vi "SRS Ramp Aux Voltage.vi"() -> ()   [LabVIEW 2020]
panel:
  in  "Channel #":i32=1 min=1 max=4 step=1
  out "Time Remaining":dbl=60.0 format="%<%H:%M:%S>t"
  out "Output Voltage":dbl format="%_4g"
  in  "Time (Hr:Min:Sec)":dbl=60.0 step=1.0 format="%<%H:%M:%S>t"
  in  "Stop Voltage":dbl=0.01 format="%_4g"
  in  "Start Ramp":bool
  in  "Cycle Time":dbl=0.1 format="%.3g"
  in  "stop":bool
  in  "VISA resource name":refnum<visa-resource-name>
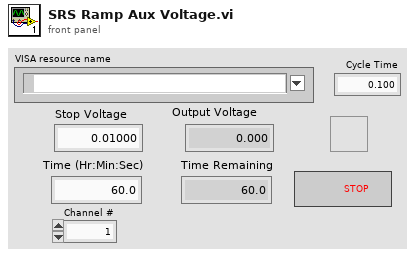
[diagram p1: front panel]
types:
  T1 = enum8{"Enabled", "Disabled", "Disabled and Grayed Out"}
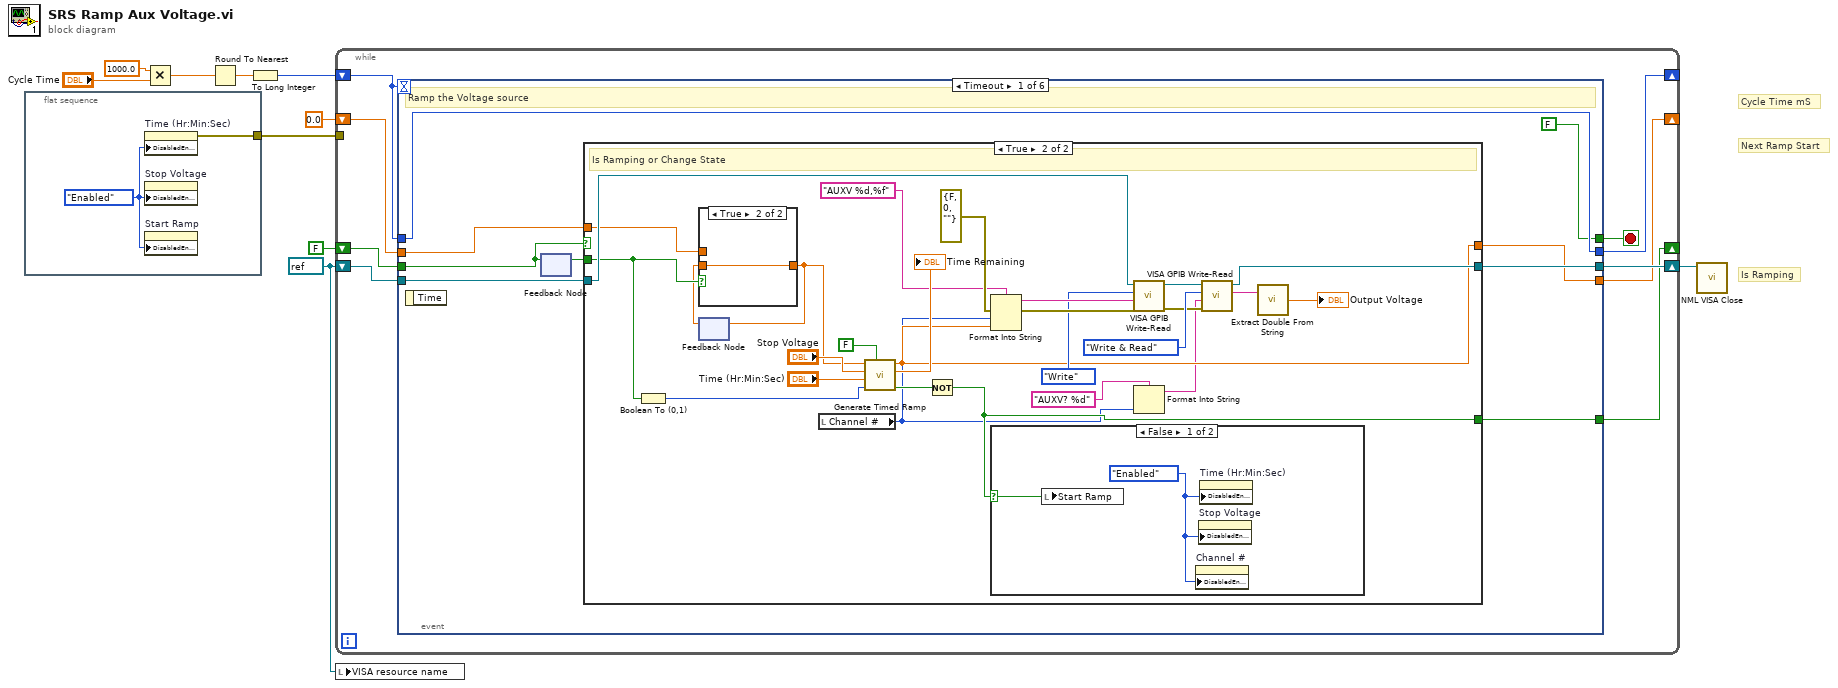
[diagram p0: block diagram]
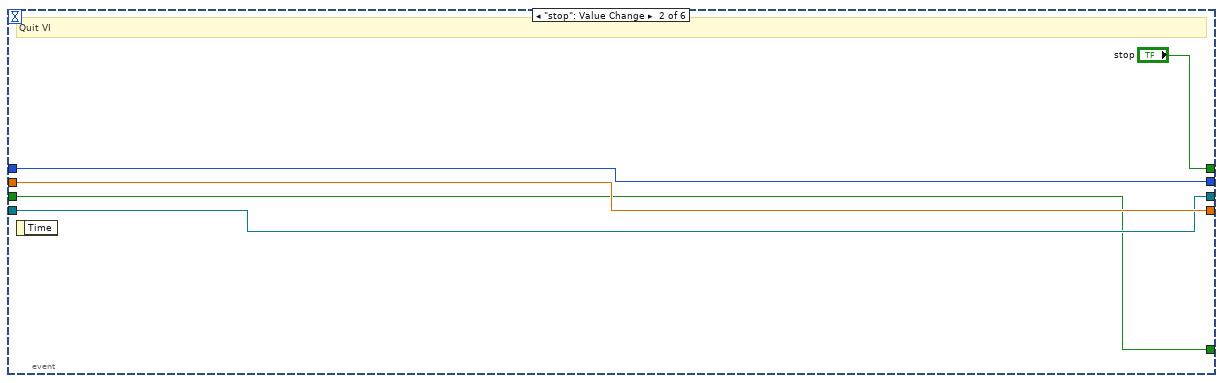
[diagram p5: hidden frame]
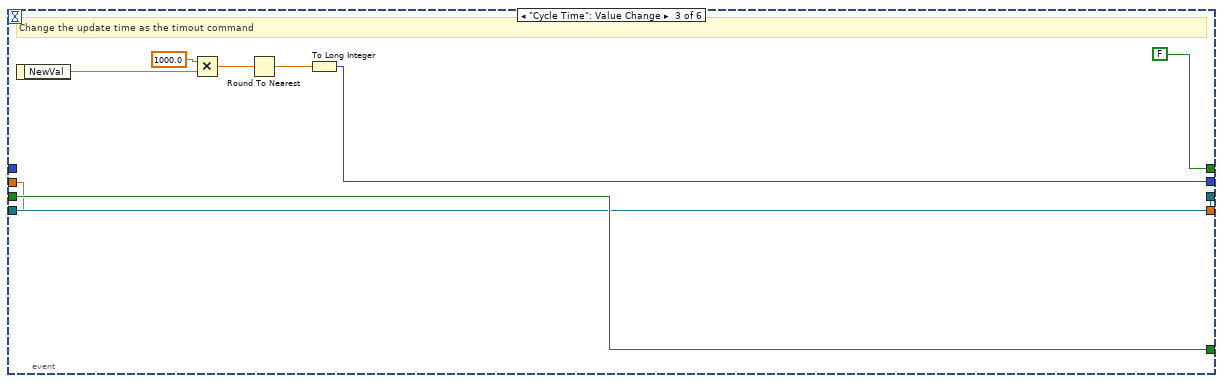
[diagram p6: hidden frame]
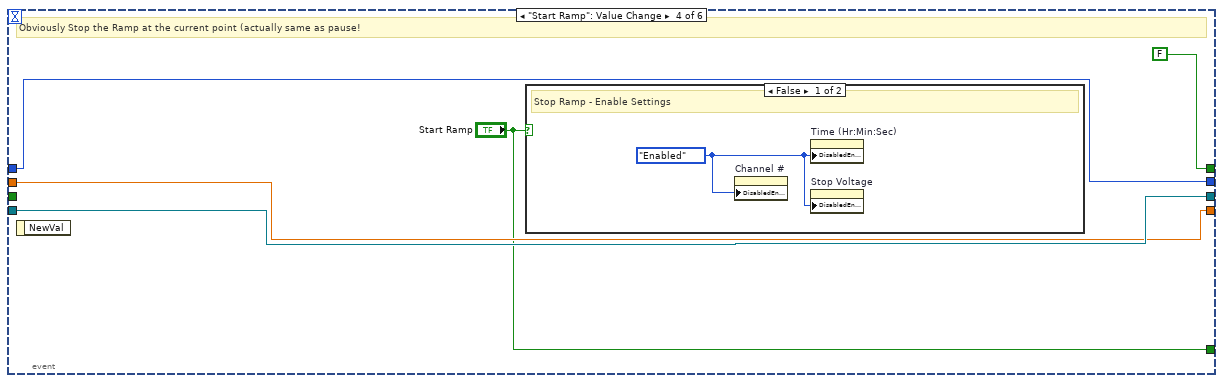
[diagram p7: hidden frame]
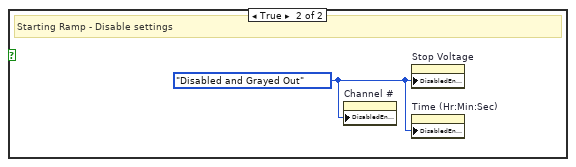
[diagram p8: hidden frame]
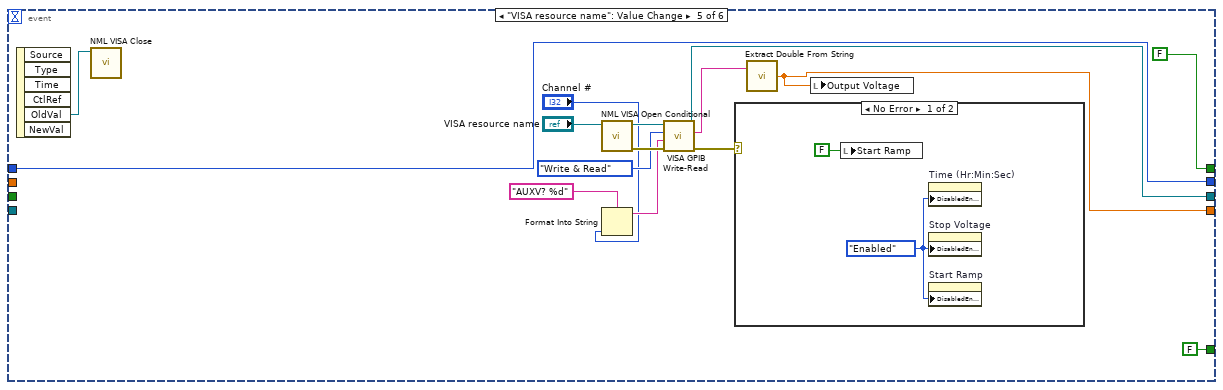
[diagram p9: hidden frame]
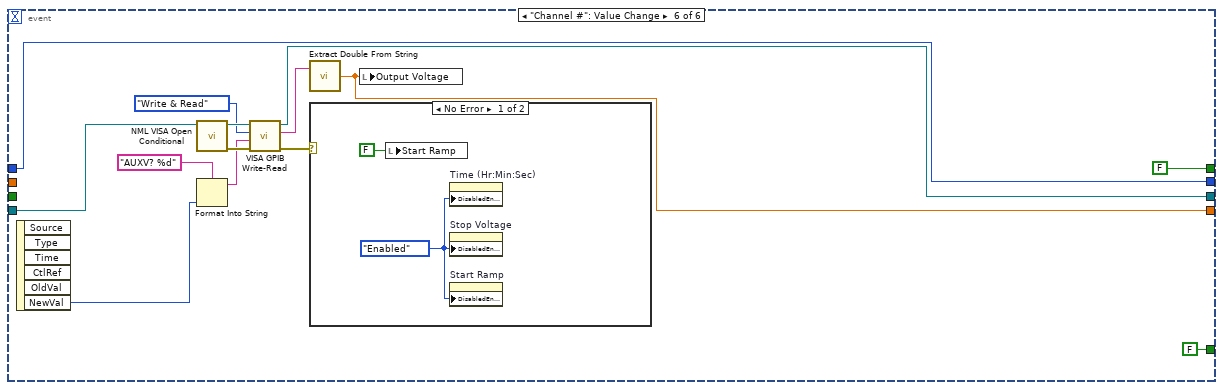
[diagram p11: hidden frame]
diagram:
  w1 = refnum<visa-resource-name> refnum ("dup VISA Session")
  # "Is Ramping"
  # "Next Ramp Start"
  # "Cycle Time mS"
  n1 = flat-sequence {
    tunnel: [w11] -> w2
    frame #0 {
      w12 = T1."Enabled" ("Disabled")
      n2 = property on="Time (Hr:Min:Sec)" class="DigNum (strict)"("DisabledEnum"=w12) -> (error out=w11:errorcluster)  [unwired: 2 in, 1 out]
      n3 = property on="Stop Voltage" class="DigNum (strict)"("DisabledEnum"=w12) -> ()  [unwired: 2 in, 2 out]
      n4 = property on="Start Ramp" class="Bool (strict)"("DisabledEnum"=w12) -> ()  [unwired: 2 in, 2 out]
    }
  }
  n5 = Multiply(x=1000.0, y="Cycle Time") -> (x*y=w9:dbl)
  n6 = Round To Nearest(number=w9) -> (nearest integer value=w7:dbl)
  n7 = To Long Integer(number=w7) -> (32bit integer=w6:i32)
  n8 = while {
    shift-right: [w17] -> w5
    shift-left: w1 -> [w18]
    shift-right: [w14] -> _
    shift-left: 0.0 ("Voitage 2450") -> [w13]
    shift-right: [w19] -> _
    shift-left: w6 -> [w20]
    shift-right: [w15] -> _
    shift-left: FALSE -> [w16]
    tunnel: w2 -> [_]
    stop <- w21 stop-if-true
    n9 = event shown="[0] Timeout" {
      selector: _ -> [_ _ _ _ _ _]
      dyn-events: _ -> [_ _ _ _ _ _]
      timeout: w20 -> [_ _ _ _ _ _]
      tunnel: [FALSE ("stop") "stop" FALSE ("stop") FALSE ("stop") FALSE ("stop") FALSE ("stop")] -> w21
      tunnel: w20 -> [w30 w68 _ w82 w96 w113]
      tunnel: [w30 w68 w74 w82 w96 w113] -> w19
      tunnel: w18 -> [w29 w66 w71 w81 _ w105]
      tunnel: [w28 w66 w71 w81 w97 w114] -> w17
      tunnel: w16 -> [w23 w65 w72 _ _ _]
      tunnel: [w26 w65 w72 "Start Ramp" FALSE ("Start Ramp") FALSE ("Start Ramp")] -> w15
      tunnel: [w24 w67 w70 w80 w93 w110] -> w14
      tunnel: w13 -> [w25 w67 w70 w80 _ _]
      event Timeout {
        # "Ramp the Voltage source"
        n10 = event-data() -> ()  [unwired: 1 in, 1 out]
        n11 = feedback-in #1(w23) -> ()
        n12 = feedback #1() -> (w22:bool)  [unwired: 1 in]
        n13 = case shown="True" w23 {
          selector: w23 -> [w31 _]
          tunnel: w29 -> [w33 w59]
          tunnel: [w33 w54] -> w28
          tunnel: [w31 w52] -> w26
          tunnel: w25 -> [w32 w50]
          tunnel: [w32 w41] -> w24
          tunnel: w22 -> [_ w51]
          frame False {
            # "Idle"
          }
          frame True {
            # "Is Ramping or Change State"
            n14 = Boolean To (0,1)(Boolean=w51) -> (0, 1=w58:i16)
            n15 = feedback #2() -> (w48:dbl)  [unwired: 1 in]
            n16 = case shown="True" w51 {
              tunnel: w50 -> [w61 _]
              tunnel: [w61 w62] -> w49
              tunnel: w48 -> [_ w62]
              frame False {
              }
              frame True {
              }
            }
            n17 = feedback-in #2(w49) -> ()
            n18 = local read "Channel #"() -> (w34:i32)
            n19 = call "Generate Timed Ramp.vi"("Log"=FALSE, "Point #"=w58, "Time (Hr:Min:Sec)"="Time (Hr:Min:Sec)", "Stop"="Stop Voltage", "Start"=w49) -> ("Stop"=w57:bool, "Time Remaining"=→"Time Remaining":dbl, "Output"=w41:dbl)  [unwired: 1 out]
            n20 = Not(x=w57) -> (.not. x?=w52:bool)
            n21 = Format Into String(format string="AUXV %d,%f" ("Command"), error in=errorcluster {"status"=FALSE, "code"=0, "source"=""} ("error in (no error)"), w34, w41) -> (resulting string=w44:string, error out=w45:errorcluster)  [unwired: 1 in]
            n22 = case shown="False" w52 {
              selector: w52 -> [w64 _]
              frame False {
                w63 = T1."Enabled" ("Disabled")
                n23 = local write "Start Ramp"(w64) -> ()
                n24 = property on="Channel #" class="DigNum (strict)"("DisabledEnum"=w63) -> ()  [unwired: 2 in, 2 out]
                n25 = property on="Stop Voltage" class="DigNum (strict)"("DisabledEnum"=w63) -> ()  [unwired: 2 in, 2 out]
                n26 = property on="Time (Hr:Min:Sec)" class="DigNum (strict)"("DisabledEnum"=w63) -> ()  [unwired: 2 in, 2 out]
              }
              frame True {
              }
            }
            n27 = call "VISA GPIB Write-Read.vi"("error in (no error)"=w45, "Command"=w44, "Action"=enum16{"Write", "Read", "Write & Read"}."Write", "VISA resource name"=w59) -> ("error out"=w37:errorcluster, "dup VISA Session"=w36:refnum<visa-resource-name>)  [unwired: 4 in, 2 out]
            n28 = Format Into String(format string="AUXV? %d" ("Command"), w34) -> (resulting string=w35:string)  [unwired: 2 in, 1 out]
            n29 = call "VISA GPIB Write-Read.vi"("error in (no error)"=w37, "Command"=w35, "Action"=enum16{"Write", "Read", "Write & Read"}."Write & Read", "VISA resource name"=w36) -> ("String Returned"=w38:string, "dup VISA Session"=w54:refnum<visa-resource-name>)  [unwired: 4 in, 2 out]
            n30 = call "Extract Double From String.vi"("string"=w38) -> ("floating pt. number"=→"Output Voltage":dbl)  [unwired: 1 in, 2 out]
          }
        }
      }
      event "stop": Value Change {
        # "Quit VI"
        n31 = event-data() -> ()  [unwired: 1 in, 1 out]
      }
      event "Cycle Time": Value Change {
        # "Change the update time as the timout command"
        n32 = event-data() -> ("NewVal"=w75:dbl)  [unwired: 1 in]
        n33 = Multiply(x=1000.0, y=w75) -> (x*y=w76:dbl)
        n34 = Round To Nearest(number=w76) -> (nearest integer value=w78:dbl)
        n35 = To Long Integer(number=w78) -> (32bit integer=w74:i32)
      }
      event "Start Ramp": Value Change {
        # "Obviously Stop the Ramp at the current point (actually same as pause!"
        n36 = event-data() -> ()  [unwired: 1 in, 1 out]
        n37 = case shown="False" "Start Ramp" {
          frame False {
            w84 = T1."Enabled" ("Disabled")
            # "Stop Ramp - Enable Settings"
            n38 = property on="Channel #" class="DigNum (strict)"("DisabledEnum"=w84) -> ()  [unwired: 2 in, 2 out]
            n39 = property on="Time (Hr:Min:Sec)" class="DigNum (strict)"("DisabledEnum"=w84) -> ()  [unwired: 2 in, 2 out]
            n40 = property on="Stop Voltage" class="DigNum (strict)"("DisabledEnum"=w84) -> ()  [unwired: 2 in, 2 out]
          }
          frame True {
            w85 = T1."Disabled and Grayed Out" ("Disabled")
            # "Starting Ramp - Disable settings"
            n41 = property on="Channel #" class="DigNum (strict)"("DisabledEnum"=w85) -> ()  [unwired: 2 in, 2 out]
            n42 = property on="Stop Voltage" class="DigNum (strict)"("DisabledEnum"=w85) -> ()  [unwired: 2 in, 2 out]
            n43 = property on="Time (Hr:Min:Sec)" class="DigNum (strict)"("DisabledEnum"=w85) -> ()  [unwired: 2 in, 2 out]
          }
        }
      }
      event "VISA resource name": Value Change {
        n44 = event-data() -> ("OldVal"=w87:refnum<visa-resource-name>)  [unwired: 1 in, 5 out]
        n45 = call "NML VISA Close.vi"("VISA resource name"=w87) -> ()  [unwired: 10 in, 1 out]
        n46 = call "NML VISA Open Conditional.vi"("VISA resource name"="VISA resource name") -> ("error out"=w100:errorcluster, "dup VISA Session"=w99:refnum<visa-resource-name>)  [unwired: 8 in, 1 out]
        n47 = Format Into String(format string="AUXV? %d" ("Command"), "Channel #") -> (resulting string=w89:string)  [unwired: 2 in, 1 out]
        n48 = call "VISA GPIB Write-Read.vi"("error in (no error)"=w100, "Command"=w89, "Action"=enum16{"Write", "Read", "Write & Read"}."Write & Read", "VISA resource name"=w99) -> ("error out"=w94:errorcluster, "String Returned"=w90:string, "dup VISA Session"=w97:refnum<visa-resource-name>)  [unwired: 4 in, 1 out]
        n49 = case shown="No Error" w94 {
          frame No Error {
            w102 = T1."Enabled" ("Disabled")
            n50 = local write "Start Ramp"(FALSE ("Start Ramp")) -> ()
            n51 = property on="Time (Hr:Min:Sec)" class="DigNum (strict)"("DisabledEnum"=w102) -> ()  [unwired: 2 in, 2 out]
            n52 = property on="Stop Voltage" class="DigNum (strict)"("DisabledEnum"=w102) -> ()  [unwired: 2 in, 2 out]
            n53 = property on="Start Ramp" class="Bool (strict)"("DisabledEnum"=w102) -> ()  [unwired: 2 in, 2 out]
          }
          frame Error {
          }
        }
        n54 = call "Extract Double From String.vi"("string"=w90) -> ("floating pt. number"=w93:dbl)  [unwired: 1 in, 2 out]
        n55 = local write "Output Voltage"(w93) -> ()
      }
      event "Channel #": Value Change {
        n56 = event-data() -> ("NewVal"=w104:i32)  [unwired: 1 in, 5 out]
        n57 = call "NML VISA Open Conditional.vi"("VISA resource name"=w105) -> ("error out"=w116:errorcluster, "dup VISA Session"=w115:refnum<visa-resource-name>)  [unwired: 8 in, 1 out]
        n58 = Format Into String(format string="AUXV? %d" ("Command"), w104) -> (resulting string=w106:string)  [unwired: 2 in, 1 out]
        n59 = call "VISA GPIB Write-Read.vi"("error in (no error)"=w116, "Command"=w106, "Action"=enum16{"Write", "Read", "Write & Read"}."Write & Read", "VISA resource name"=w115) -> ("error out"=w111:errorcluster, "String Returned"=w107:string, "dup VISA Session"=w114:refnum<visa-resource-name>)  [unwired: 4 in, 1 out]
        n60 = call "Extract Double From String.vi"("string"=w107) -> ("floating pt. number"=w110:dbl)  [unwired: 1 in, 2 out]
        n61 = case shown="No Error" w111 {
          frame No Error {
            w118 = T1."Enabled" ("Disabled")
            n62 = local write "Start Ramp"(FALSE ("Start Ramp")) -> ()
            n63 = property on="Time (Hr:Min:Sec)" class="DigNum (strict)"("DisabledEnum"=w118) -> ()  [unwired: 2 in, 2 out]
            n64 = property on="Stop Voltage" class="DigNum (strict)"("DisabledEnum"=w118) -> ()  [unwired: 2 in, 2 out]
            n65 = property on="Start Ramp" class="Bool (strict)"("DisabledEnum"=w118) -> ()  [unwired: 2 in, 2 out]
          }
          frame Error {
          }
        }
        n66 = local write "Output Voltage"(w110) -> ()
      }
    }
  }
  n67 = local write "VISA resource name"(w1) -> ()
  n68 = call "NML VISA Close.vi"("VISA resource name"=w5) -> ()  [unwired: 10 in, 1 out]
